vi "Waveformgraph.vi"(2 "Save Current Image":bool, 3 "Waveform Graph":dbl[][](graph)) -> (0 "error out":errorcluster, 1 "Match":bool)   [LabVIEW 2011]
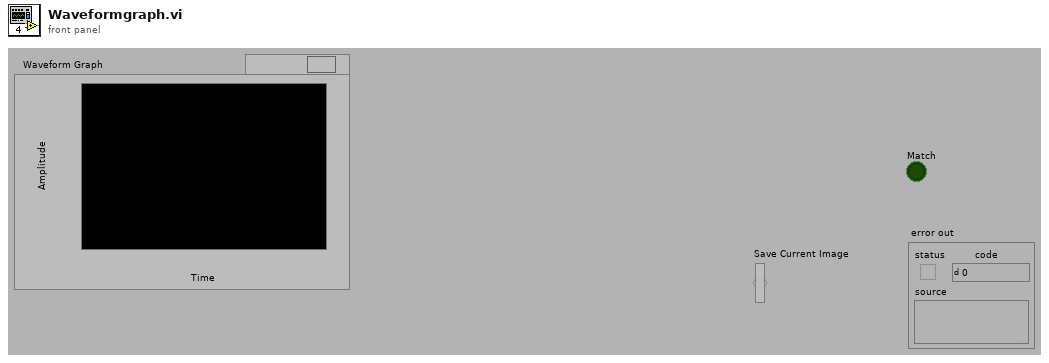
[diagram p1: front panel]
types:
  T1 = enum16{"open", "open or create", "create or replace", "create", "open (read only)"}
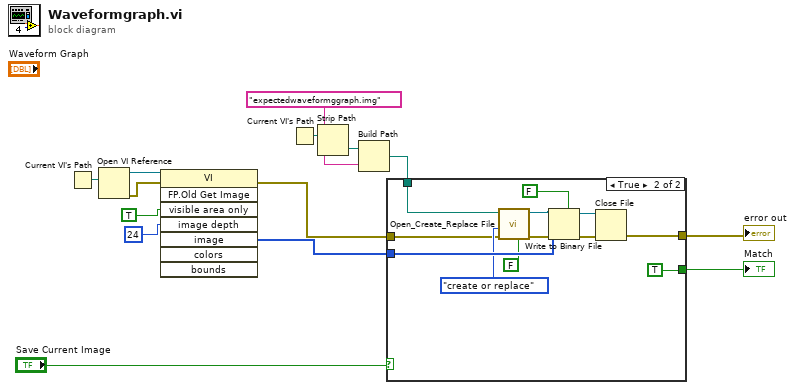
[diagram p0: block diagram]
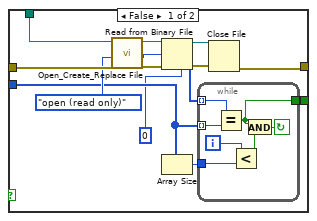
[diagram p2: hidden frame]
diagram:
  n1 = Current VI's Path() -> (path=w14:path)
  n2 = Open VI Reference(vi path=w14) -> (vi reference=w11:refnum<vi>, error out=w10:errorcluster)  [unwired: 1 in, 4 out]
  n3 = invoke class="VI" method="FP.Old Get Image"(reference=w11, error in=w10, "visible area only"=TRUE, "image depth"=24) -> (error out=w7:errorcluster, "image"=w8:u8[])  [unwired: 4 in, 6 out]
  n4 = Current VI's Path() -> (path=w4:path)
  n5 = Strip Path(path=w4) -> (stripped path=w5:path)  [unwired: 1 out]
  n6 = Build Path(base path=w5, name or relative path="expectedwaveformggraph.img") -> (appended path=w2:path)
  n7 = case shown="True" "Save Current Image" {
    tunnel: w8 -> [w17 w45]
    tunnel: w7 -> [w27 w41]
    tunnel: [w21 w40] -> w6
    tunnel: w2 -> [w28 w39]
    tunnel: [w18 TRUE] -> w1
    frame False {
      n8 = call <vilib>:"Open_Create_Replace File.vi"("error in (no error)"=w27, "function (open:0)"=T1."open (read only)", "file path"=w28) -> ("error out"=w23:errorcluster, "file size (bytes)"=w15:i32, "refnum"=w22:refnum<file>)  [unwired: 3 in, 3 out]
      n9 = Read from Binary File(5:u8 0, 8:w23, 10:w15, 11:w22) -> (0:w25:errorcluster, 2:w20:u8[], 3:w24:refnum<file>)  [unwired: 3 out]
      n10 = Array Size(array=w17) -> (size(s)=w19:i32)
      n11 = while {
        tunnel: w20 -> [w34] mode=indexing
        tunnel: w17 -> [w35] mode=indexing
        tunnel: w19 -> [w30]
        tunnel: [w29] -> w18
        i -> [w31]
        stop <- w33 continue-if-true
        n12 = Equal?(x=w34, y=w35) -> (x = y?=w29:bool)
        n13 = Less?(x=w31, y=w30) -> (x < y?=w32:bool)
        n14 = And(x=w29, y=w32) -> (x .and. y?=w33:bool)
      }
      n15 = Close File(refnum=w24, error in=w25) -> (error out=w21:errorcluster)  [unwired: 1 out]
    }
    frame True {
      n16 = call <vilib>:"Open_Create_Replace File.vi"("advisory dialog? (display:T)"=FALSE, "error in (no error)"=w41, "function (open:0)"=T1."create or replace", "file path"=w39) -> ("error out"=w46:errorcluster, "refnum"=w47:refnum<file>)  [unwired: 3 in, 3 out]
      n17 = Write to Binary File(file (use dialog)=w47, data=w45, error in=w46, 5:FALSE ("prepend array or string size? (T)")) -> (refnum out=w42:refnum<file>, error out=w43:errorcluster)  [unwired: 3 out]
      n18 = Close File(refnum=w42, error in=w43) -> (error out=w40:errorcluster)  [unwired: 1 out]
    }
  }
  "error out" <- w6
  "Match" <- w1
